vi "Parse Line.vi"(11 "format string":string) -> (3 "array type (2D Dbl)":string[](array[string]))   [LabVIEW 2019, in "Day 8.lvlib"]
uses:
  Day 8.lvlib
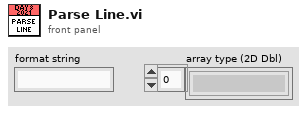
[diagram p1: front panel]
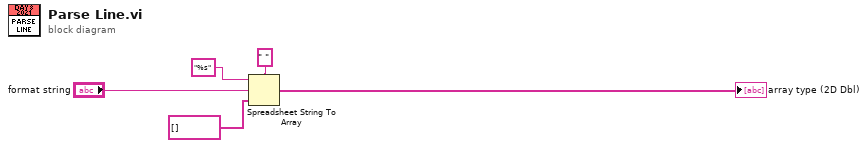
[diagram p0: block diagram]
diagram:
  n1 = Spreadsheet String To Array(delimiter (Tab)=" ", format string="%s", spreadsheet string="format string", array type (2D Dbl)=string[] []) -> (array=→"array type (2D Dbl)":string[])
